vi "Variant to String.vi"(8 "error in":errorcluster, 9 "Variant Value":variant) -> (0 "error out":errorcluster, 1 "String Value":string)   [LabVIEW 2018, in "Tag Engine.lvlib"]
uses:
  Tag Engine.lvlib
  <vilib>/Utility/Data Type/NI_Data Type.lvlib
  <vilib>/JDP Science/JSONtext/JSONtext.lvlib
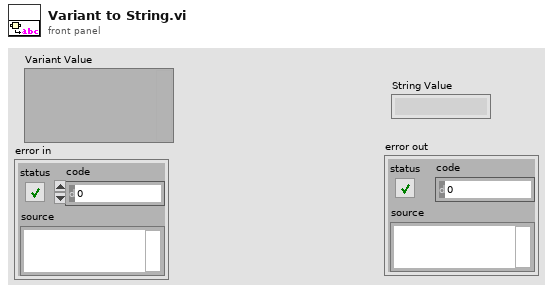
[diagram p1: front panel]
types:
  T1 = typedef "NI_Data Type.lvlib/Data Type.ctl" = enum8{"Invalid Type", "Void", "I8", "I16", "I32", "I64", "U8", "U16", "U32", "U64", "Single Float", "Double Float", "Extended Float", "Single Complex", "Double Complex", "Extended Complex", "Enum U8", "Enum U16", "Enum U32", "Enum U64", "Single Float With Unit", "Double Float With Unit", "Extended Float With Unit", "Single Complex with Unit", "Double Complex with Unit", "Extended Complex with Unit", "Boolean", "String", "Path", "Picture", "Tag", "Array", "Cluster", "Variant", "LV Variant", "Waveform", "Timestamp", "Digital Waveform", "Digital Data", "ExpressData", "Refnum", "External Data", "VI", "Poly VI", "LabVIEW Class Instance", "Fixed Point"}
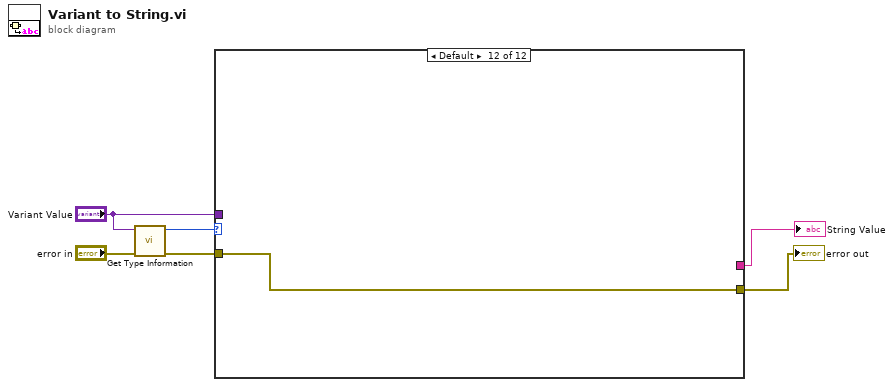
[diagram p0: block diagram]
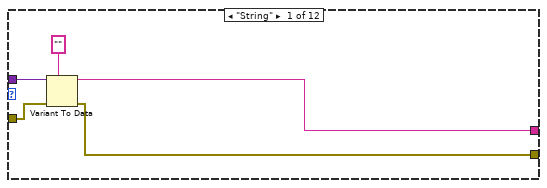
[diagram p2: hidden frame]
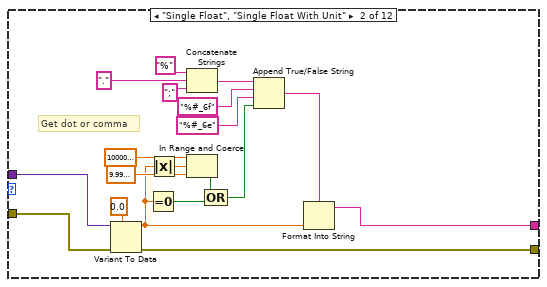
[diagram p3: hidden frame]
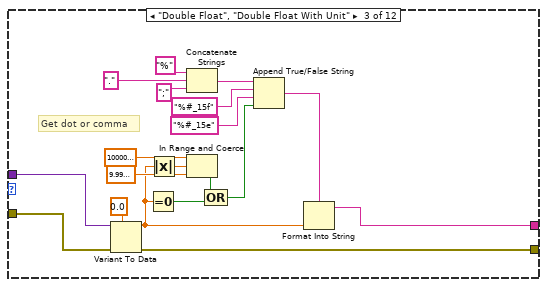
[diagram p4: hidden frame]
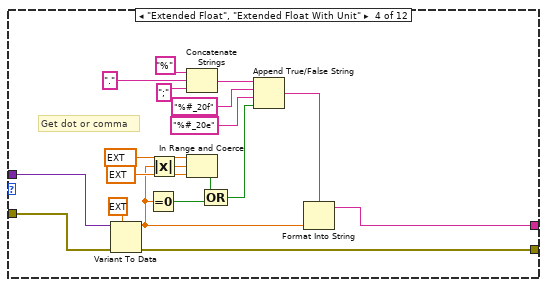
[diagram p5: hidden frame]
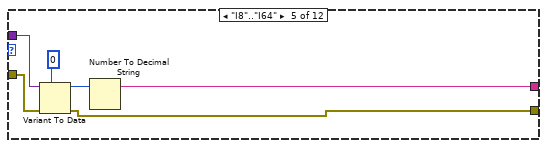
[diagram p6: hidden frame]
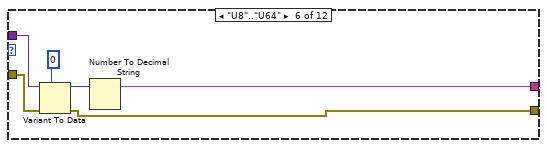
[diagram p7: hidden frame]
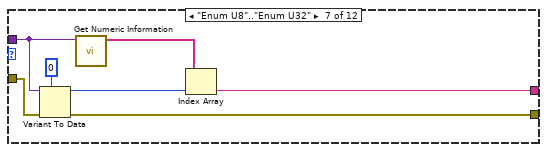
[diagram p8: hidden frame]
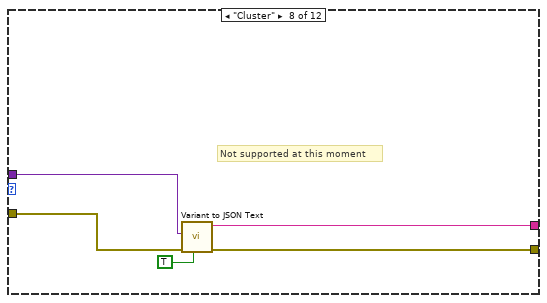
[diagram p9: hidden frame]
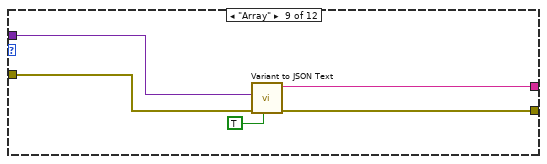
[diagram p10: hidden frame]
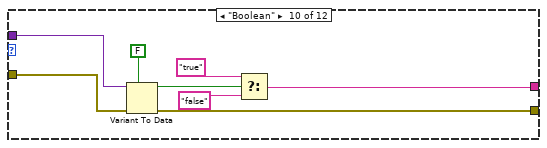
[diagram p11: hidden frame]
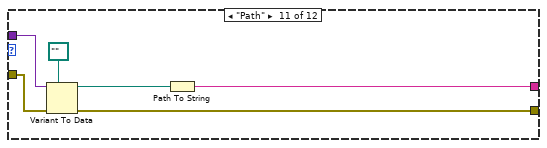
[diagram p12: hidden frame]
diagram:
  n1 = call <vilib>:"Get Type Information.vi"("error in (no error)"="error in", "Variant"="Variant Value") -> ("error out"=w3:errorcluster, "Type"=w5:T1)  [unwired: 5 in, 3 out]
  n2 = case shown="Default" w5 {
    tunnel: [w9 w16 w35 w54 w72 w78 w81 w91 w95 w103 w109 _] -> w1
    tunnel: "Variant Value" -> [w10 w15 w34 w52 w71 w77 w84 w92 w97 w100 w108 _]
    tunnel: w3 -> [w8 w14 w33 w51 w70 w76 w83 w90 w93 w99 w107 w112]
    tunnel: [w7 w13 w31 w50 w69 w75 w82 w89 w94 w98 w106 w112] -> w2
    frame "String" {
      n3 = Variant To Data(error in=w8, type="" ("Format String"), Variant=w10) -> (data=w9:string, error out=w7:errorcluster)
    }
    frame "Single Float", "Single Float With Unit" {
      # "Get dot or comma"
      n4 = Variant To Data(error in=w14, type=sgl 0.0, Variant=w15) -> (data=w26:sgl, error out=w13:errorcluster)
      n5 = Equal To 0?(x=w26) -> (x = 0?=w25:bool)
      n6 = Absolute Value(x=w26) -> (abs(x)=w27:sgl)
      n7 = Concatenate Strings("%" ("format string"), ".", ";" ("format string")) -> (w21:string)
      n8 = In Range and Coerce(upper limit=sgl 1000000.0, x=w27, lower limit=sgl 0.0001 ("upper limit")) -> (In Range?=w24:bool)  [unwired: 1 out]
      n9 = Compound Arithmetic op=OR(w24, w25) -> (w18:bool)
      n10 = Append True/False String(1:w18, 2:"%#_6e" ("format string"), 3:"%#_6f" ("format string"), 4:w21) -> (0:w17:string)
      n11 = Format Into String(format string=w17, w26) -> (resulting string=w16:string)  [unwired: 2 in, 1 out]
    }
    frame "Double Float", "Double Float With Unit" {
      # "Get dot or comma"
      n12 = Variant To Data(error in=w33, type=0.0, Variant=w34) -> (data=w45:dbl, error out=w31:errorcluster)
      n13 = Equal To 0?(x=w45) -> (x = 0?=w44:bool)
      n14 = Absolute Value(x=w45) -> (abs(x)=w46:dbl)
      n15 = Concatenate Strings("%" ("format string"), "." ("string"), ";" ("format string")) -> (w40:string)
      n16 = In Range and Coerce(upper limit=1000000.0, x=w46, lower limit=9.999999747378752e-05 ("upper limit")) -> (In Range?=w43:bool)  [unwired: 1 out]
      n17 = Compound Arithmetic op=OR(w43, w44) -> (w37:bool)
      n18 = Append True/False String(1:w37, 2:"%#_15e" ("format string"), 3:"%#_15f" ("format string"), 4:w40) -> (0:w36:string)
      n19 = Format Into String(format string=w36, w45) -> (resulting string=w35:string)  [unwired: 2 in, 1 out]
    }
    frame "Extended Float", "Extended Float With Unit" {
      # "Get dot or comma"
      n20 = Variant To Data(error in=w51, type=ext 0.0, Variant=w52) -> (data=w64:ext, error out=w50:errorcluster)
      n21 = Equal To 0?(x=w64) -> (x = 0?=w63:bool)
      n22 = Absolute Value(x=w64) -> (abs(x)=w65:ext)
      n23 = Concatenate Strings("%" ("format string"), "." ("string"), ";" ("format string")) -> (w59:string)
      n24 = In Range and Coerce(upper limit=ext 1000000.0, x=w65, lower limit=ext 9.999999747378752e-05 ("upper limit")) -> (In Range?=w62:bool)  [unwired: 1 out]
      n25 = Compound Arithmetic op=OR(w62, w63) -> (w56:bool)
      n26 = Append True/False String(1:w56, 2:"%#_20e" ("format string"), 3:"%#_20f" ("format string"), 4:w59) -> (0:w55:string)
      n27 = Format Into String(format string=w55, w64) -> (resulting string=w54:string)  [unwired: 2 in, 1 out]
    }
    frame "I8".."I64" {
      n28 = Variant To Data(error in=w70, type=i64 0, Variant=w71) -> (data=w73:i64, error out=w69:errorcluster)
      n29 = Number To Decimal String(number=w73) -> (decimal integer string=w72:string)  [unwired: 1 in]
    }
    frame "U8".."U64" {
      n30 = Variant To Data(error in=w76, type=u64 0, Variant=w77) -> (data=w79:u64, error out=w75:errorcluster)
      n31 = Number To Decimal String(number=w79) -> (decimal integer string=w78:string)  [unwired: 1 in]
    }
    frame "Enum U8".."Enum U32" {
      n32 = Variant To Data(error in=w83, type=0, Variant=w84) -> (data=w86:i32, error out=w82:errorcluster)
      n33 = call <vilib>:"Get Numeric Information.vi"("Variant"=w84) -> ("Enum Names"=w85:string[])  [unwired: 7 in, 3 out]
      n34 = Index Array(array=w85, index=w86) -> (element=w81:string)
    }
    frame "Cluster" {
      # "Not supported at this moment"
      n35 = call <vilib>:"Variant to JSON Text.vi"("Pretty Print?"=TRUE, "error in (no error)"=w90, "Variant"=w92) -> ("error out"=w89:errorcluster, "<JSON>"=w91:string)  [unwired: 6 in, 1 out]
    }
    frame "Array" {
      n36 = call <vilib>:"Variant to JSON Text.vi"("Pretty Print?"=TRUE, "error in (no error)"=w93, "Variant"=w97) -> ("error out"=w94:errorcluster, "<JSON>"=w95:string)  [unwired: 6 in, 1 out]
    }
    frame "Boolean" {
      n37 = Variant To Data(error in=w99, type=FALSE, Variant=w100) -> (data=w104:bool, error out=w98:errorcluster)
      n38 = Select(t="true", s=w104, f="false") -> (s? t:f=w103:string)
    }
    frame "Path" {
      n39 = Variant To Data(error in=w107, type=path "" ("Format String"), Variant=w108) -> (data=w110:path, error out=w106:errorcluster)
      n40 = Path To String(path=w110) -> (string=w109:string)
    }
    frame Default {
    }
  }
  "String Value" <- w1
  "error out" <- w2
